vi "subAddRules.vi"(8 "error in (no error)":errorcluster, 9 "Rules":T1, 11 "CDependencyInspector in":refnum<class "CDependencyInspection.lvclass">) -> (0 "error out":errorcluster, 3 "CDependencyInspector out":refnum<class "CDependencyInspection.lvclass">)   [LabVIEW 2020, in "DependencyInspection.lvlib" / "CDependencyInspection.lvclass"]
uses:
  CDependencyInspection.lvclass
  LabVIEWObjectFactory/LabVIEWObjectFactory.lvlib
  CRuleList/CRuleList.lvclass
  LabVIEWObjectInterfaces/IDependencyItemRule/IDependencyItemRule.lvclass
  E:/Repos/LVDependencyInspector/obj/Addons/LabVIEWObjectInterfaces.lvlibp/LabVIEWObjectInterfaces/IDependencyItemRule/IDependencyItemRule.lvclass
  E:/Repos/LVDependencyInspector/obj/Addons/LabVIEWObjectInterfaces.lvlibp/LabVIEWObjectInterfaces/ILabVIEWItem/ILabVIEWItem.lvclass
  ExtensionInterfaces/IRuleFileParser/RulesDefinition.ctl
  ExtensionInterfaces/IRuleFileParser/IRuleFileParser.lvclass
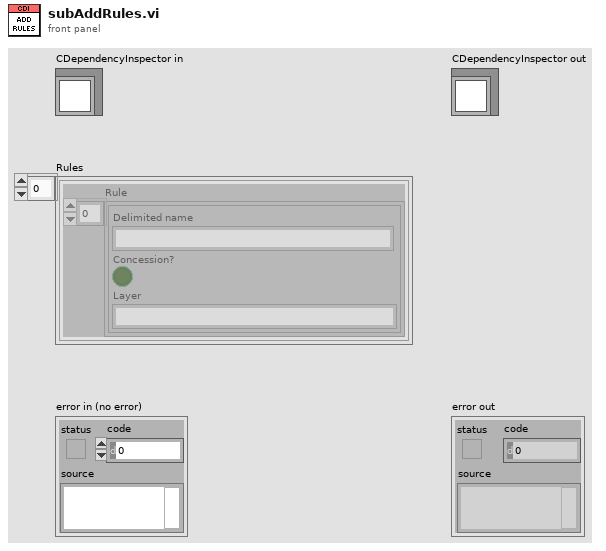
[diagram p1: front panel]
types:
  T1 = typedef "ExtensionInterfaces.lvlib/IRuleFileParser.lvclass/RulesDefinition.ctl" = cluster{"Rule":cluster{"Delimited name":string, "Concession?":bool, "Layer":string}[]}[]
  T2 = cluster{"Delimited name":string, "Concession?":bool, "Layer":string}[]
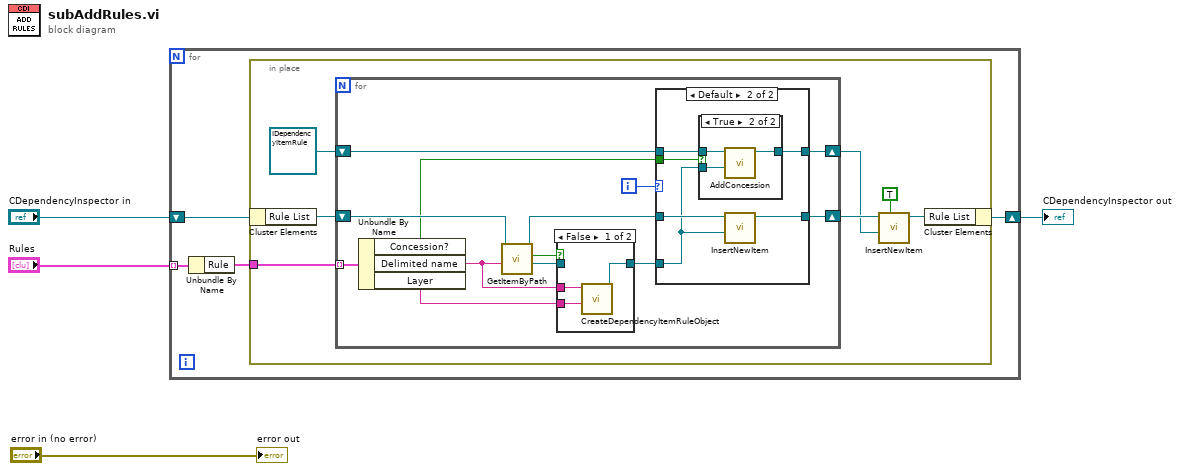
[diagram p0: block diagram]
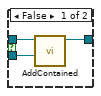
[diagram p4: hidden frame]
diagram:
  n1 = for {
    tunnel: "Rules" -> [w5] mode=indexing
    shift-right: [w7] -> w1
    shift-left: "CDependencyInspector in" -> [w8]
    n2 = Unbundle By Name(w5) -> ("Rule"=w6:T2)
    n3 = in-place {
      in-place-border: w6 -> [w15]
      n4 = in-place-cluster #1(w8) -> ("Rule List"=w10:refnum<class "CRuleList.lvclass">)
      n5 = for {
        tunnel: w15 -> [w28] mode=indexing
        shift-right: [w27] -> w12
        shift-left: w10 -> [w26]
        shift-right: [w25] -> w11
        shift-left: refnum<class "IDependencyItemRule.lvclass"> refnum ("IDependencyItemRule") -> [w24]
        i -> [w23]
        n6 = Unbundle By Name(w28) -> ("Concession?"=w18:bool, "Delimited name"=w16:string, "Layer"=w17:string)
        n7 = call-dynamic "GetItemByPath.vi"("Path"=w16, "CRuleList in"=w26) -> ("IDependencyItemRule"=w22:refnum<class "IDependencyItemRule.lvclass">, "key found?"=w21:bool, "CRuleList out"=w19:refnum<class "CRuleList.lvclass">)  [unwired: 6 in, 1 out]
        n8 = case shown="False" w21 {
          tunnel: w16 -> [w31 _]
          tunnel: [w30 w32] -> w20
          tunnel: w22 -> [_ w32]
          tunnel: w17 -> [w29 _]
          frame False {
            n9 = call "CreateDependencyItemRuleObject.vi"("Parent Layer"=w29, "delimited name"=w31) -> ("IDependencyItemRule"=w30:refnum<class "IDependencyItemRule.lvclass">)  [unwired: 8 in, 1 out]
          }
          frame True {
          }
        }
        n10 = case shown="Default" w23 {
          tunnel: [w34 w38] -> w25
          tunnel: w20 -> [w34 w36]
          tunnel: w24 -> [_ w37]
          tunnel: w19 -> [w33 w40]
          tunnel: [w33 w39] -> w27
          tunnel: w18 -> [_ w35]
          frame 0 {
          }
          frame Default {
            n11 = case shown="True" w35 {
              tunnel: [w43 w44] -> w38
              tunnel: w37 -> [w42 w46]
              tunnel: w36 -> [w41 w45]
              frame False {
                n12 = call-dynamic "AddContained.vi"("Item to contain"=w41, "ILabVIEWItem in"=w42) -> ("ILabVIEWItem out"=w43:refnum<class "IDependencyItemRule.lvclass">)  [unwired: 7 in, 2 out]
              }
              frame True {
                n13 = call-dynamic "AddConcession.vi"("Item to conceed"=w45, "IDependencyItemRule in"=w46) -> ("IDependencyItemRule out"=w44:refnum<class "IDependencyItemRule.lvclass">)  [unwired: 8 in, 1 out]
              }
            }
            n14 = call-dynamic "InsertNewItem.vi"("IDependencyRule in"=w36, "CRuleList in"=w40) -> ("CRuleList out"=w39:refnum<class "CRuleList.lvclass">)  [unwired: 7 in, 2 out]
          }
        }
      }
      n15 = call-dynamic "InsertNewItem.vi"("Replace?"=TRUE, "IDependencyRule in"=w11, "CRuleList in"=w12) -> ("CRuleList out"=w9:refnum<class "CRuleList.lvclass">)  [unwired: 6 in, 2 out]
      n16 = in-place-cluster #1("Rule List"=w9) -> (w7:refnum<class "CDependencyInspection.lvclass">)
    }
  }
  "CDependencyInspector out" <- w1
  "error out" <- "error in (no error)"
